vi "Get BLISS_Validate Save Folder.vi"(8 "error in":errorcluster, 11 "Data Parameters in":T1={"Start Time"=timestamp(3690155740.033191 s since 1904-01-01), "Save to Folder"=path "", "Forces in Theater"=[{"Force Commander"="BlissUT124", "Units"=[]}, {"Force Commander"="BlissMP146", "Units"=[]}, {"Force Commander"="BlissMP145", "Units"=[]}, {"Force Commander"="BlissMP140", "Units"=[]}, {"Force Commander"="BlissMP137", "Units"=[]}, {"Force Commander"="BlissMP135", "Units"=[]}, {"Force Commander"="BlissMP134", "Units"=[]}, {"Force Commander"="BlissMP132", "Units"=[]}, {"Force Commander"="BlissMA109", "Units"=[]}, {"Force Commander"="BlissMA107", "Units"=[]}, {"Force Commander"="BlissMA106", "Units"=[]}, {"Force Commander"="BlissMA101", "Units"=[]}, {"Force Commander"="BlissLU118", "Units"=[]}, {"Force Commander"="BlissLU117", "Units"=[]}, {"Force Commander"="BlissLU116", "Units"=[]}, {"Force Commander"="BlissLU115", "Units"=[]}, {"Force Commander"="BlissLU114", "Units"=[]}, {"Force Commander"="BlissLU113", "Units"=[]}, {"Force Commander"="BlissLU111", "Units"=[]}, {"Force Commander"="BlissLL185", "Units"=[]}, {"Force Commander"="BlissLL183", "Units"=[]}, {"Force Commander"="BlissLL173", "Units"=[]}, {"Force Commander"="BlissLL172", "Units"=[]}, {"Force Commander"="BlissLL171", "Units"=[]}, {"Force Commander"="BlissJH103", "Units"=[]}, {"Force Commander"="BlissJH102", "Units"=[]}, {"Force Commander"="BlissJH101", "Units"=[]}, {"Force Commander"="BlissJE116", "Units"=[]}, {"Force Commander"="BlissJE115", "Units"=[]}, {"Force Commander"="BlissJE114", "Units"=[]}, {"Force Commander"="BlissJE111", "Units"=[]}, {"Force Commander"="BlissHD183", "Units"=[]}, {"Force Commander"="BlissHD182", "Units"=[]}, {"Force Commander"="BlissHD181", "Units"=[]}, {"Force Commander"="BlissGPDFFPL", "Units"=[]}, {"Force Commander"="BlissEUWIPES", "Units"=[]}, {"Force Commander"="BlissEU179", "Units"=[]}, {"Force Commander"="BlissEU178", "Units"=[]}, {"Force Commander"="BlissEU177", "Units"=[]}, {"Force Commander"="Blissdvds02", "Units"=[]}, {"Force Commander"="BlissDOWIPES", "Units"=[]}, {"Force Commander"="BlissCR022", "Units"=[]}, {"Force Commander"="BlissCR021", "Units"=[]}, {"Force Commander"="BlissCG167", "Units"=[]}, {"Force Commander"="BlissCG166", "Units"=[]}, {"Force Commander"="BlissCG161", "Units"=[]}, {"Force Commander"="BlissCG160", "Units"=[]}, {"Force Commander"="BlissCG159", "Units"=[]}, {"Force Commander"="BlissCG158", "Units"=[]}, {"Force Commander"="BlissCG157", "Units"=[]}, {"Force Commander"="BlissCG156", "Units"=[]}, {"Force Commander"="BlissCG151", "Units"=[]}, {"Force Commander"="BlissCB172", "Units"=[]}, {"Force Commander"="BlissCB171", "Units"=[]}, {"Force Commander"="BlissCB108", "Units"=[]}, {"Force Commander"="BlissCB107", "Units"=[]}, {"Force Commander"="BlissBV181", "Units"=[]}, {"Force Commander"="BlissBV162", "Units"=[]}, {"Force Commander"="BlissAK177", "Units"=[]}, {"Force Commander"="BlissAK176", "Units"=[]}, {"Force Commander"="BlissAK175", "Units"=[]}, {"Force Commander"="BlissAK174", "Units"=[]}, {"Force Commander"="BlissAK173", "Units"=[]}, {"Force Commander"="BlissAK172", "Units"=[]}, {"Force Commander"="BlissAK171", "Units"=[]}, {"Force Commander"="BlissAK139", "Units"=[]}, {"Force Commander"="BlissAK134", "Units"=[]}, {"Force Commander"="BlissAK131", "Units"=[]}, {"Force Commander"="BlissAH163", "Units"=[]}, {"Force Commander"="BlissAH162", "Units"=[]}, {"Force Commander"="BlissAH161", "Units"=[]}, {"Force Commander"="BlissAH122", "Units"=[]}, {"Force Commander"="BlissAH121", "Units"=[]}, {"Force Commander"="BlissAD106", "Units"=[]}, {"Force Commander"="BlissAD104", "Units"=[]}, {"Force Commander"="BlissAB105", "Units"=[]}, {"Force Commander"="BlissAB104", "Units"=[]}]}) -> (0 "error out":errorcluster, 2 "Valid Folder":bool, 3 "Enable/Disable":T8(ring))   [LabVIEW 2020]
uses:
  Get BLISS_Global Error Codes.vi
  MC5e Squad_Info.ctl
  MC5e Unit_Status_List.ctl
  MC5e Data_Parameters.ctl
  MC5e Terrain types.ctl
  Location.ctl
  MC5e Unit.ctl
  MC5e Force.ctl
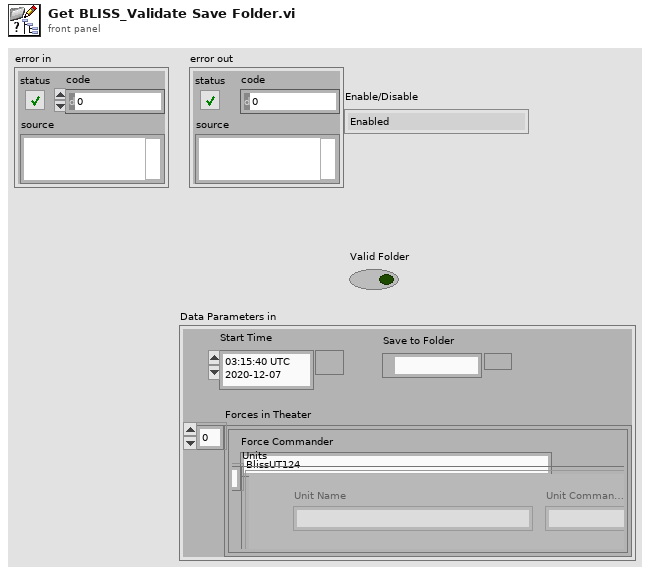
[diagram p1: front panel]
types:
  T1 = typedef "MC5e Data_Parameters.ctl" = cluster{"Start Time":timestamp, "Save to Folder":path, "Forces in Theater":T2[]}
  T2 = typedef "MC5e Force.ctl" = cluster{"Force Commander":string, "Units":T3[]}
  T3 = typedef "MC5e Unit.ctl" = cluster{"Squad List":T4, "Unit Fatigue Level":enum16{"Not Fatigued", "Fatigued", "Seriously Fatigued"}, "Flying Unit":bool, "Mounted Unit":bool, "Difficult Terrain Types":T6, "Full BR":dbl, "Defending from Stronghold":bool, "Speed":dbl, "Capacity %":dbl, "Morale":dbl, "Current BR":dbl, "Location":T7, "Unit Name":string, "Unit Commander":string, "Unit Notes":string}
  T4 = typedef "MC5e Unit_Status_List.ctl" = T5[]
  T5 = typedef "MC5e Squad_Info.ctl" = cluster{"Squad Name":string, "# Soldiers":dbl, "Battle Rating":dbl, "Flying":bool, "Mounted":bool, "Speed":dbl, "Range":dbl, "Morale":dbl, "Token Image":variant, "Max Endurance":dbl, "Current Endurance":dbl, "Difficult Terrain":T6}
  T6 = typedef "MC5e Terrain types.ctl" = cluster{"Artic / snow / ice)":bool, "Coast":bool, "Desert / sand":bool, "Forest / woodland":bool, "Grassland / plains":bool, "Mountain / canyons":bool, "Underdark / caverns":bool, "Acquatic / rivers, lakes, ocean":bool}
  T7 = typedef "Location.ctl" = cluster{"X coordinate":dbl, "Y coordinate":dbl}
  T8 = enum8{"Enabled", "Disabled", "Disabled and Grayed Out"}
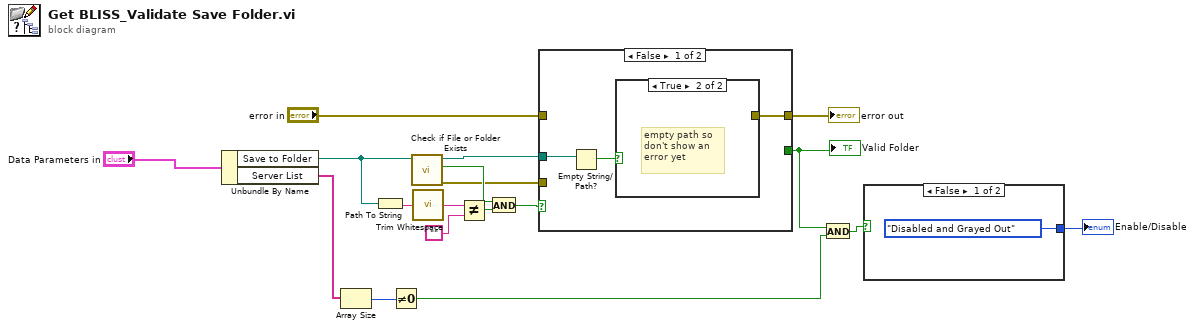
[diagram p0: block diagram]
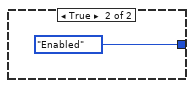
[diagram p2: hidden frame]
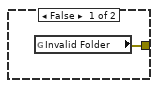
[diagram p3: hidden frame]
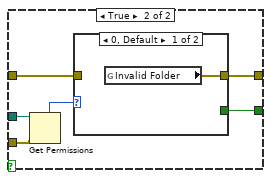
[diagram p4: hidden frame]
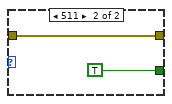
[diagram p5: hidden frame]
diagram:
  n1 = Unbundle By Name("Data Parameters in") -> ("Save to Folder"=w10:path, "Server List"=w4:string[])
  n2 = Array Size(array=w4) -> (size(s)=w3:i32)
  n3 = Path To String(path=w10) -> (string=w13:string)
  n4 = Not Equal To 0?(x=w3) -> (x != 0?=w1:bool)
  n5 = call <vilib>:"Check if File or Folder Exists.vi"("path"=w10) -> ("error out"=w11:errorcluster, "file or folder exists?"=w17:bool, "dup path"=w12:path)  [unwired: 8 in]
  n6 = call <vilib>:"Trim Whitespace.vi"("string"=w13) -> ("trimmed string"=w14:string)  [unwired: 1 in]
  n7 = Not Equal?(x=w14, y="") -> (x != y?=w16:bool)
  n8 = And(x=w17, y=w16) -> (x .and. y?=w18:bool)
  n9 = case shown="False" w18 {
    tunnel: w11 -> [_ w28]
    tunnel: w12 -> [w20 w27]
    tunnel: [_ w25] -> w8
    tunnel: [w21 w24] -> w6
    tunnel: "error in" -> [_ w23]
    frame False {
      n10 = Empty String/Path?(string/path=w20) -> (empty?=w19:bool)
      n11 = case shown="True" w19 {
        tunnel: [w22 _] -> w21
        frame False {
          n12 = global read "Get BLISS_Global Error Codes.vi" "Invalid Folder"() -> (w22:errorcluster)
        }
        frame True {
          # "empty path so \ndon't show an \nerror yet"
        }
      }
    }
    frame True {
      n13 = Get Permissions(8:w28, 11:w27) -> (5:w26:i16)  [unwired: 4 out]
      n14 = case shown="0, Default" w26 {
        tunnel: [_ TRUE] -> w25
        tunnel: [w29 w30] -> w24
        tunnel: w23 -> [_ w30]
        frame 0, Default {
          n15 = global read "Get BLISS_Global Error Codes.vi" "Invalid Folder"() -> (w29:errorcluster)
        }
        frame 511 {
        }
      }
    }
  }
  "Valid Folder" <- w8
  "error out" <- w6
  n16 = And(x=w8, y=w1) -> (x .and. y?=w2:bool)
  n17 = case shown="False" w2 {
    tunnel: [T8."Disabled and Grayed Out" ("Disabled") T8."Enabled" ("Disabled")] -> w9
    frame False {
    }
    frame True {
    }
  }
  "Enable/Disable" <- w9
